vi "Initialize.vi"(8 "error in (no error)":errorcluster, 10 "Array of Motors":refnum<class "Motor.lvclass">[](array[class]), 11 "MotionSystem in":refnum<class "MotionSystem.lvclass">) -> (0 "error out":errorcluster, 2 "duplicate labels?":bool, 3 "MotionSystem out":refnum<class "MotionSystem.lvclass">)   [LabVIEW 2016, in "MotionSystem.lvlib" / "MotionSystem.lvclass"]
uses:
  <userlib>/Common Components/Hardware/Abstract System/MotionSystem/MotionSystem/MotionSystem.lvclass
  <userlib>/Common Components/Hardware/Motor/Motor/Motor.lvclass
  C:/Program Files (x86)/National Instruments/LabVIEW 2016/user.lib/Common Components/Hardware/Abstract Hardware/Hardware.lvclass
  <userlib>/Common Components/Hardware/Abstract Hardware/Hardware.lvclass/Hardware.ctl
  <userlib>/Common Components/Hardware/Abstract System/MotionSystem/MotionSystem/MotionSystem.lvclass/MotionSystem.ctl
  <userlib>/Common Components/Hardware/Abstract Hardware/Read Label.vi
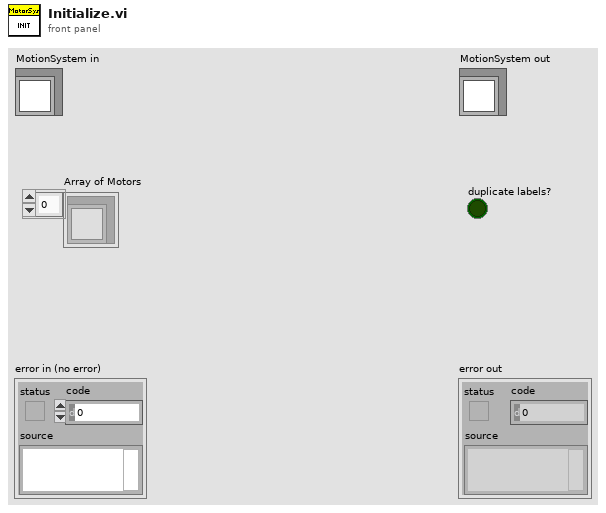
[diagram p1: front panel]
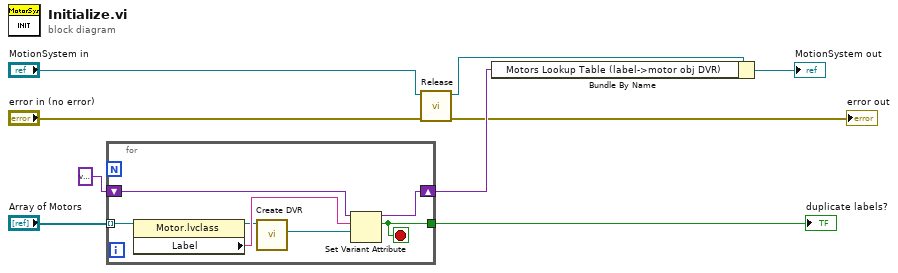
[diagram p0: block diagram]
diagram:
  n1 = for {
    tunnel: "Array of Motors" -> [w12] mode=indexing
    shift-right: [w15] -> w5
    shift-left: variant -> [w16]
    tunnel: [w13] -> w7
    stop <- w13 stop-if-true
    n2 = property class="Motor.lvclass"(reference=w12) -> (reference out=w11:refnum<class "Motor.lvclass">, "Label"=w14:string)  [unwired: 1 in, 1 out]
    n3 = call <userlib>:"Create DVR.vi"("Motor in"=w11) -> ("data value reference"=w10:refnum<data-value>)  [unwired: 8 in, 2 out]
    n4 = Set Variant Attribute(Variant=w16, name=w14, value=w10) -> (Variant out=w15:variant, replaced=w13:bool)  [unwired: 1 in, 1 out]
  }
  "duplicate labels?" <- w7
  n5 = call <userlib>:"Release.vi"("error in (no error)"="error in (no error)", "MotionSystem in"="MotionSystem in") -> ("error out"=→"error out":errorcluster, "MotionSystem out"=w3:refnum<class "MotionSystem.lvclass">)  [unwired: 8 in]
  n6 = Bundle By Name(cluster=w3, "Motors Lookup Table (label->motor obj DVR)"=w5) -> (→"MotionSystem out":refnum<class "MotionSystem.lvclass">)
